vi "Format Full Endpoint Name.vi"(11 "Full Endpoint Name":string) -> (3 "Formatted Endpoint Name":string)   [LabVIEW 2020, in "Routing and Faulting System Explorer.lvlib"]
uses:
  Routing and Faulting System Explorer.lvlib
  <vilib>/regexp/Match Regular Expression.xnode
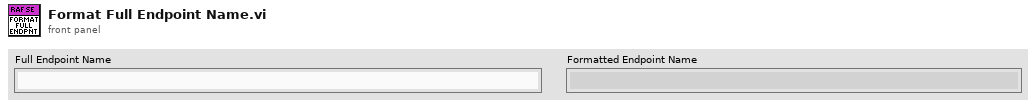
[diagram p1: front panel]
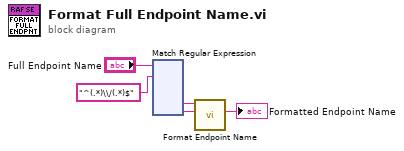
[diagram p0: block diagram]
diagram:
  n1 = xnode "Match Regular Expression"("input string"="Full Endpoint Name", "regular expression"="^(.*)\\/(.*)$" ("search string")) -> ("submatch 1"=w4:string, "submatch 2"=w3:string)  [unwired: 4 in, 5 out]
  n2 = call "Format Endpoint Name.vi"("Endpoint"=w3, "Module Path"=w4) -> ("Formatted Endpoint Name"=→"Formatted Endpoint Name":string)  [unwired: 8 in, 1 out]
